vi "Delete DVR_Notifier.vi"(0 "data value reference":refnum<data-value>, 11 "error in (no error)":errorcluster) -> (15 "error out":errorcluster)   [LabVIEW 2020, in "Data Communication Transmitter.lvlib" / "Notifiers.lvclass"]
doc: "Delete DVR notifier"
uses:
  Classes/Children/Intra-Application/Children/With Data/Children/Notifiers/Notifiers.lvclass
  Classes/Children/Intra-Application/Children/With Data/Children/Notifiers/Notifiers.lvclass/Notifiers.ctl
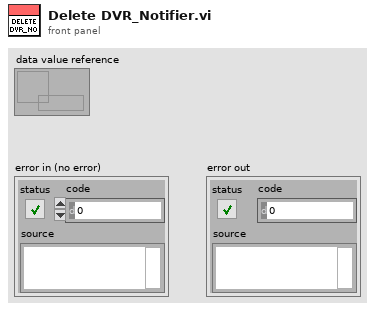
[diagram p1: front panel]
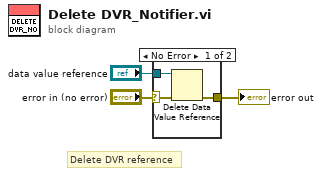
[diagram p0: block diagram]
diagram:
  # "Delete DVR reference"
  n1 = case shown="No Error" "error in (no error)" {
    selector: "error in (no error)" -> [w5 w7]
    tunnel: [w6 w7] -> w3
    tunnel: "data value reference" -> [w4 _]
    frame No Error {
      n2 = Delete Data Value Reference(data value reference=w4, error in=w5) -> (error out=w6:errorcluster)  [unwired: 1 out]
    }
    frame Error {
    }
  }
  "error out" <- w3
